vi "error - not unique.vi"(8 "error in (no error)":errorcluster) -> (0 "error out":errorcluster)   [LabVIEW 2024, in "status manager.lvlib"]
uses:
  status manager.lvlib
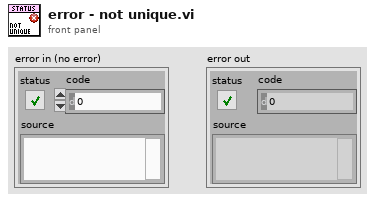
[diagram p1: front panel]
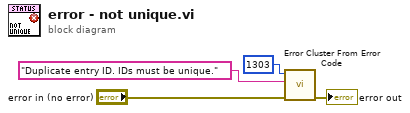
[diagram p0: block diagram]
diagram:
  n1 = call <vilib>:"Error Cluster From Error Code.vi"("error in (no error)"="error in (no error)", "error message (\"\")"="Duplicate entry ID. IDs must be unique.", "error code (0)"=1303) -> ("error out"=→"error out":errorcluster)  [unwired: 6 in]
